vi "Write time.vi"(8 "error in (no error)":errorcluster, 10 "time / date":timestamp, 11 "Test Results in":refnum<class "Test Results.lvclass">) -> (0 "error out":errorcluster, 3 "Test Results out":refnum<class "Test Results.lvclass">)   [LabVIEW 2020, in "Test Results.lvclass"]
uses:
  Test Results.lvclass
  Test Results.lvclass/Test Results.ctl
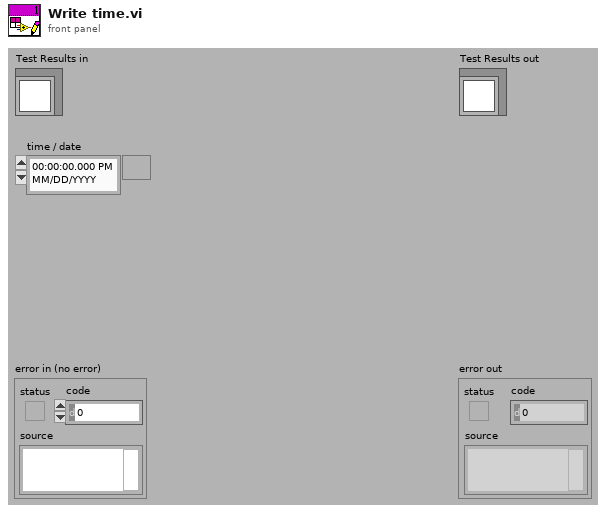
[diagram p1: front panel]
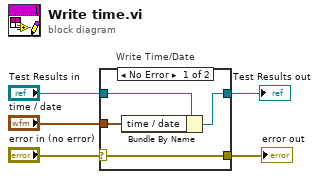
[diagram p0: block diagram]
diagram:
  # "Write Time/Date"
  n1 = case shown="No Error" "error in (no error)" {
    selector: "error in (no error)" -> [w9 w10]
    tunnel: [w9 w10] -> w4
    tunnel: [w7 w11] -> w2
    tunnel: "Test Results in" -> [w8 w11]
    tunnel: "time / date" -> [w6 _]
    frame No Error {
      n2 = Bundle By Name(cluster=w8, "time / date"=w6) -> (w7:refnum<class "Test Results.lvclass">)
    }
    frame Error {
    }
  }
  "error out" <- w4
  "Test Results out" <- w2
